vi "Toggle Button.vi"(2 "Button":bool, 3 "State":enum16{"PRESSED ON", "ON", "PRESSED OFF", "OFF"}(ring)) -> (0 "Output":bool, 1 "State Output":enum16{"PRESSED ON", "ON", "PRESSED OFF", "OFF"}(ring))   [LabVIEW 2020]
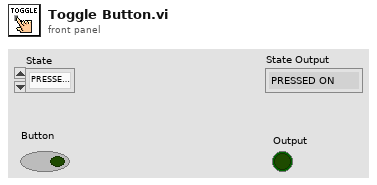
[diagram p1: front panel]
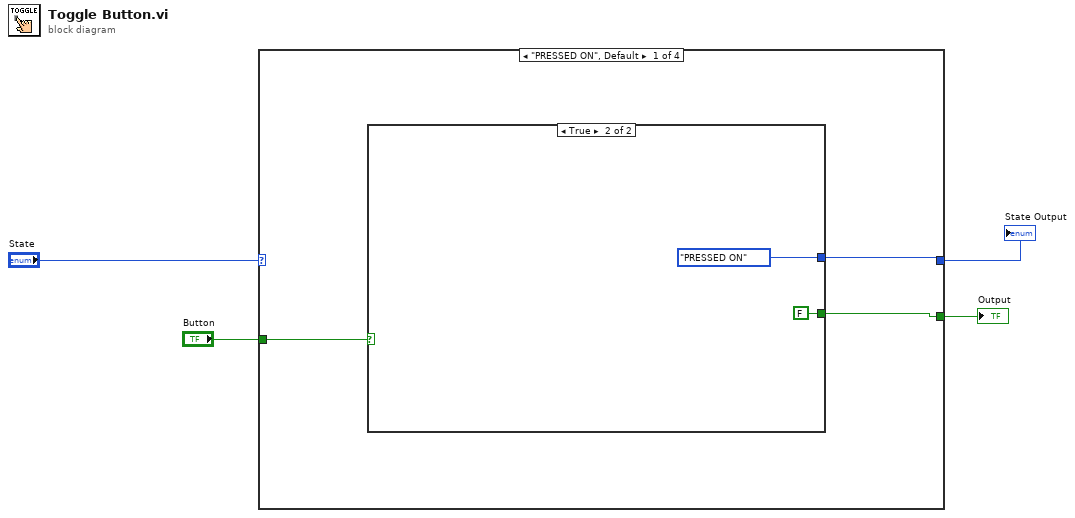
[diagram p0: block diagram]
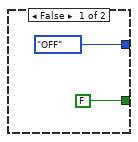
[diagram p2: hidden frame]
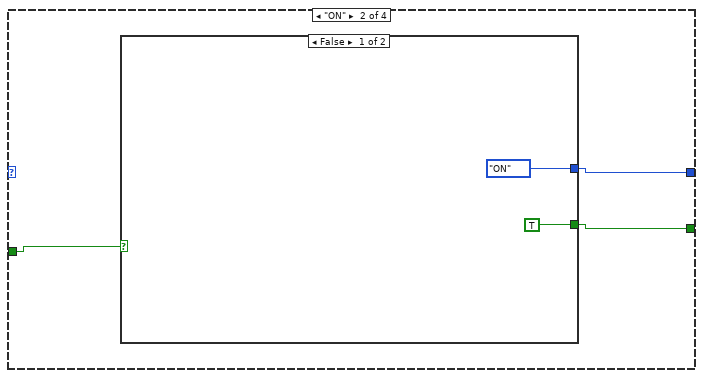
[diagram p3: hidden frame]
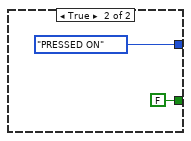
[diagram p4: hidden frame]
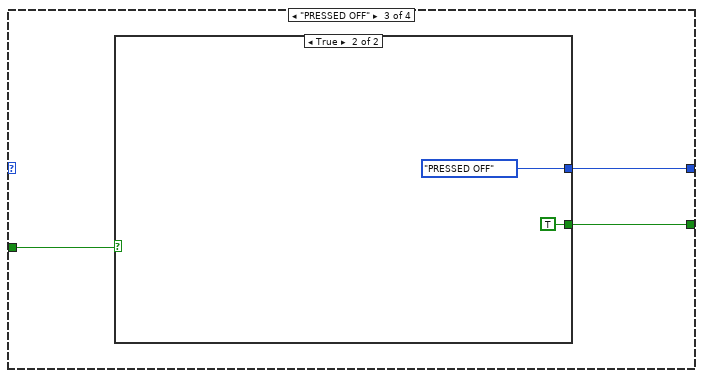
[diagram p5: hidden frame]
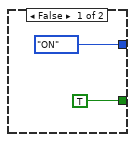
[diagram p6: hidden frame]
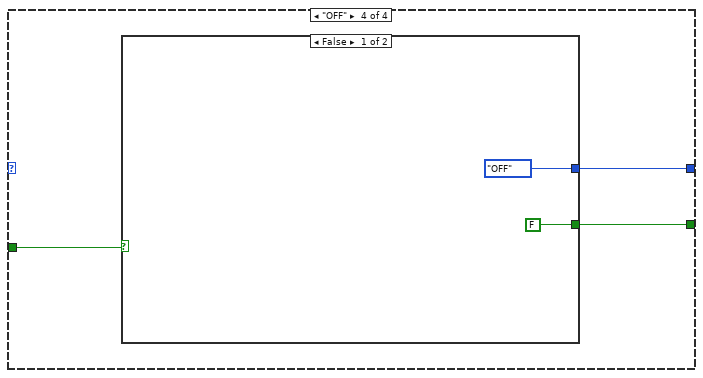
[diagram p7: hidden frame]
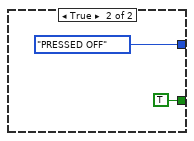
[diagram p8: hidden frame]
diagram:
  n1 = case shown="\"PRESSED ON\", Default" "State" {
    tunnel: "Button" -> [w5 w14 w19 w28]
    tunnel: [w6 w12 w20 w27] -> w2
    tunnel: [w7 w13 w21 w26] -> w1
    frame "PRESSED ON", Default {
      n2 = case shown="True" w5 {
        tunnel: [FALSE FALSE] -> w6
        tunnel: [enum16{"PRESSED ON", "ON", "PRESSED OFF", "OFF"}."OFF" ("State") enum16{"PRESSED ON", "ON", "PRESSED OFF", "OFF"}."PRESSED ON" ("State")] -> w7
        frame False {
        }
        frame True {
        }
      }
    }
    frame "ON" {
      n3 = case shown="False" w14 {
        tunnel: [TRUE FALSE] -> w12
        tunnel: [enum16{"PRESSED ON", "ON", "PRESSED OFF", "OFF"}."ON" ("State") enum16{"PRESSED ON", "ON", "PRESSED OFF", "OFF"}."PRESSED ON" ("State")] -> w13
        frame False {
        }
        frame True {
        }
      }
    }
    frame "PRESSED OFF" {
      n4 = case shown="True" w19 {
        tunnel: [TRUE TRUE] -> w20
        tunnel: [enum16{"PRESSED ON", "ON", "PRESSED OFF", "OFF"}."ON" ("State") enum16{"PRESSED ON", "ON", "PRESSED OFF", "OFF"}."PRESSED OFF" ("State")] -> w21
        frame False {
        }
        frame True {
        }
      }
    }
    frame "OFF" {
      n5 = case shown="False" w28 {
        tunnel: [FALSE TRUE] -> w27
        tunnel: [enum16{"PRESSED ON", "ON", "PRESSED OFF", "OFF"}."OFF" ("State") enum16{"PRESSED ON", "ON", "PRESSED OFF", "OFF"}."PRESSED OFF" ("State")] -> w26
        frame False {
        }
        frame True {
        }
      }
    }
  }
  "Output" <- w2
  "State Output" <- w1
